vi "Main.vi"() -> ()   [LabVIEW 2017, in "Client.lvlib"]
uses:
  Client.lvlib
  UI_API/UIReferences.ctl
  UI_API/SR Fields.ctl
  ParserSorter/SR Data.ctl
  ParserSorter/AE Group.ctl
  ParserSorter/SR Status.ctl
  ParserSorter/SR Level.ctl
  ParserSorter/SR Type.ctl
  ServerCommunications/TypeDefs/Connection Status.ctl
  CommunicationsFrameWork/TypeDefs/InternalData.ctl
  ServerCommunications/TypeDefs/SR List.ctl
  ServerCommunications/TypeDefs/SR Data.ctl
  ClientErrorHandler/ErrorLoopInitData.ctl
  CommunicationsFrameWork/CommsFrameWork.lvlib
  ServerCommunications/CommsServer.lvlib
  <vilib>/httpClient/LabVIEWHTTPClient.lvlib
  ClientErrorHandler/ClientErrorHandler.lvlib
  ClientLogger/ClientLogger.lvlib
  ParserSorter/ParserSorter.lvlib
  UI_API/UI_API.lvlib
panel:
  in  "Filter Preset":enum16{"All", "Eastern Europe", "DACH"}(ring)
  out "Time to Refresh":dbl(slide) scale=0.0..10.0
  in  "Stop":bool
  out "Connection Quality":dbl(knob) scale=0.0..10.0
  out "Connected?":bool
  out "Last Update":timestamp
  in  "Refresh":bool
  in  "AE Level":enum16{"AE / ELP", "AE Intern"}(ring)
  in  "AE Groups":i32[](listbox)
  in  "SRs Tab":enum32{"Unassigned", "Assigned", "Debug"}(tab)
  out "Unassigned Sorted SRs":string[][](table)
  out "Assigned Sorted SRs":string[][](table)
  out "Last Error":errorcluster
  in  "Text":string="Manual Log Entry"
  in  "Type":string="Event"
  in  "Generate Log Entry":bool
  in  "Injected Error":errorcluster
  in  "Generate Error":bool
  out "Header":string="HTTP/1.1 200 OK\r\nConnection: Keep-Alive\r\nServer: Embedthis-http\r\nContent-Type: text/xml; charset=utf-8\r\nCache-Control: no-cache\r\nDate: Fri, 26 Jan 2018 14:34:54 GMT\r\nContent-Length: 21\r\nKeep-Alive: timeout=60, max=199\r\n\r\n"
  out "Body":string="<Response></Response>"
  in  "DecorationControl":i32(listbox)
  # "Heartbeat Communication"
  # "Manual Loop Control"
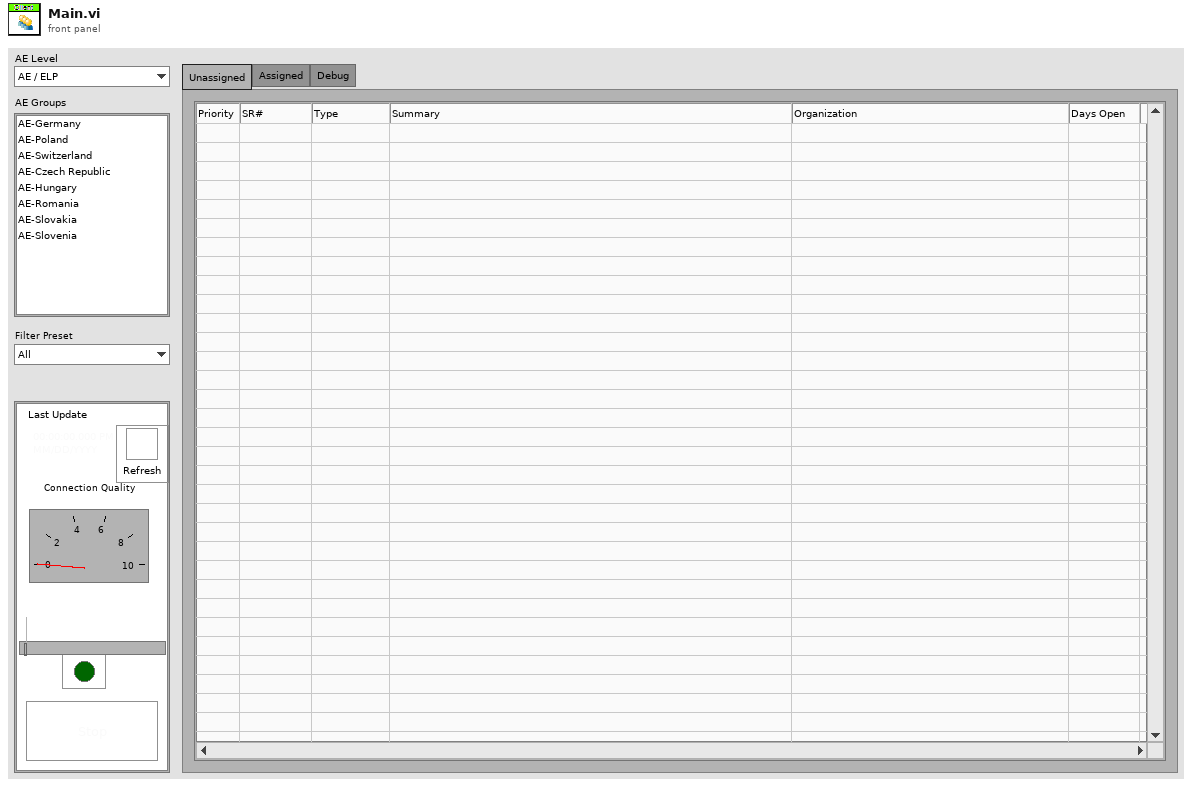
[diagram p1: front panel]
types:
  T1 = typedef "Client.lvlib/CommsFrameWork.lvlib/CommReferences.ctl" = cluster{"ErrorEventReg":refnum<event-registration>, "ErrorEvent":refnum<user-event>, "Queues":cluster{"MHLClient":refnum<queue>, "ErrorHandler":refnum<queue>, "EventHandler":refnum<queue>, "ConnectionHandler":refnum<queue>, "UIHandler":refnum<queue>, "Logger":refnum<queue>}}
  T2 = typedef "LVPoint32TypeDef.ctl" = cluster{"Horizontal":i32, "Vertical":i32}
  T3 = typedef "Client.lvlib/UI_API.lvlib/UIReferences.ctl" = cluster{"Assigned SRs":refnum<vi>, "Unassigned SRs":refnum<vi>, "AE Level":refnum<vi>, "AE Groups":refnum<vi>}
  T4 = typedef "Client.lvlib/ParserSorter.lvlib/SR Data.ctl" = cluster{"SR Number":i64, "AE Group":T5, "SR Owner":string, "Summary":string, "SR Status":T6, "Days Open":dbl, "Prio":T7, "SR Type":T8, "Service Level":string, "Last Updated":timestamp, "First Name":string, "Last Name":string, "Organisation Name":string, "Creation Date":timestamp, "Needs Merging?":bool, "English Flag?":bool}
  T5 = typedef "Client.lvlib/ParserSorter.lvlib/AE Group.ctl" = enum32{"NaN", "AE-Germany", "AE-Poland", "AE-Switzerland", "AE-Czech Republic", "AE-Hungary", "AE-Romania", "AE-Slovakia", "AE-Slovenia"}
  T6 = typedef "Client.lvlib/ParserSorter.lvlib/SR Status.ctl" = enum32{"NaN", "Caller Abandoned", "Created in Error", "Declined to Purchase Support", "Expired", "Forum Resolved AE", "Forum Resolved Customer", "IN WORK", "IN WORK Collab with AES", "IN WORK Collab with PSE", "IN WORK Collab with SE", "IN WORK Escalation", "IN WORK Customer Added Note", "Open", "Potentially Resolved", "POC Resolved", "Resolved", "RMA Waiting on Customer", "RMA Open", "RMA In Progress", "RMA Closed - DOA", "RMA Closed", "RMA Approved for Return", "Project Complete", "Presumed Resolved", "IN WORK Wait on Customer"}
  T7 = typedef "Client.lvlib/ParserSorter.lvlib/SR Level.ctl" = enum16{"Prio 1", "Prio 2", "Prio 3", "Prio 4"}
  T8 = typedef "Client.lvlib/ParserSorter.lvlib/SR Type.ctl" = enum32{"NaN", "ATE Core Configurations (BYOATE)", "Activation", "BioBench", "CAN", "CM C Series", "Calibration", "Consulting Services", "CounterTimer", "DAQExpress", "DASYLab", "DIAdem", "DMM", "DSA HW", "Digital_IO", "FIRST (NIC Only)", "FieldBus", "FieldPoint", "Functional Savety", "GATI", "GPIB", "HMI and Industrial PCs", "HiQ", "HighSpeedDigital_IO", "IMAQ", "IOTech Vibration", "Industrial Communications", "InsightCM", "LV", "LV CD&Sim", "LV Comms", "LV Controls Add-Ons", "LV Embedded", "LV MathScript RT", "LV NXG", "LV NXT", "LVDSC", "LVFPGA", "LVPDA and LV Touch Panel", "LVRT", "LabWindows_CVI", "Lookout", "MATRIXx", "MStudioDotNet", "MStudioVisualBasic", "MStudioVisualC", "Measure (Legacy)", "Motion", "MultifunctionDAQ", "Multimedia Test HW/SW", "Multisim (EWB)", "NI Update Service", "OPC Servers", "Optical (OSI)", "PXI Controllers, Chassis, MXI", "PXI Timing and Sync", "Power Supplies and SMUs", "Powertrain Controls", "RAID", "RF", "RF Software", "RIO", "SC Express", "SCC", "SCXI", "SPEEDY-33 (Hyperception)", "STS", "ScopeDigitizers", "Serial", "Signal Sources", "SignalCondOther", "SignalExpress", "Software Defined Intruments", "Sound and Vibration SW", "Switch Executive", "Switches", "TestStand", "USRP", "Ultiboard (EWB)", "VBench", "VI Logger", "VXI_MXI", "VeriStand", "VisionSW", "VolumeLicenseMgr", "WSN", "Web UI Builder", "myRIO"}
  T9 = typedef "Client.lvlib/CommsServer.lvlib/Connection Status.ctl" = cluster{"Connection Quality":dbl, "Last Update":timestamp}
  T10 = typedef "Client.lvlib/ParserSorter.lvlib/SR Fields.ctl" = enum16{"SR Number", "AE Group", "SR Owner", "Summary", "SR Status", "Days Open", "Prio", "SR Type", "Service Level", "Last Updated", "First Name", "Last Name", "Organisation Name", "Creation Date", "Needs Merging?", "English Flag?"}
  T11 = typedef "Client.lvlib/ClientErrorHandler.lvlib/ErrorLoopInitData.ctl" = cluster{"ErrorsToIgnore":i32[]}
  T12 = typedef "Client.lvlib/CommsFrameWork.lvlib/InternalData.ctl" = cluster{"Connection Data":cluster{"IP":string, "Port":string, "ClientName":string}}
  T13 = typedef "Client.lvlib/CommsServer.lvlib/SR List.ctl" = T14[]
  T14 = typedef "Client.lvlib/CommsServer.lvlib/SR Data.ctl" = cluster{"SR#":dbl, "Group":string, "Owner":string, "Problem Summary":string, "Last Updated":timestamp, "Customer First Name":string, "Customer Last Name":string, "Company":string, "Created On":timestamp, "SR Type":string, "Status":string, "Service Level":string, "Channel":string, "Days Open":dbl}
  T15 = cluster{"IP":string, "Port":string, "ClientName":string}
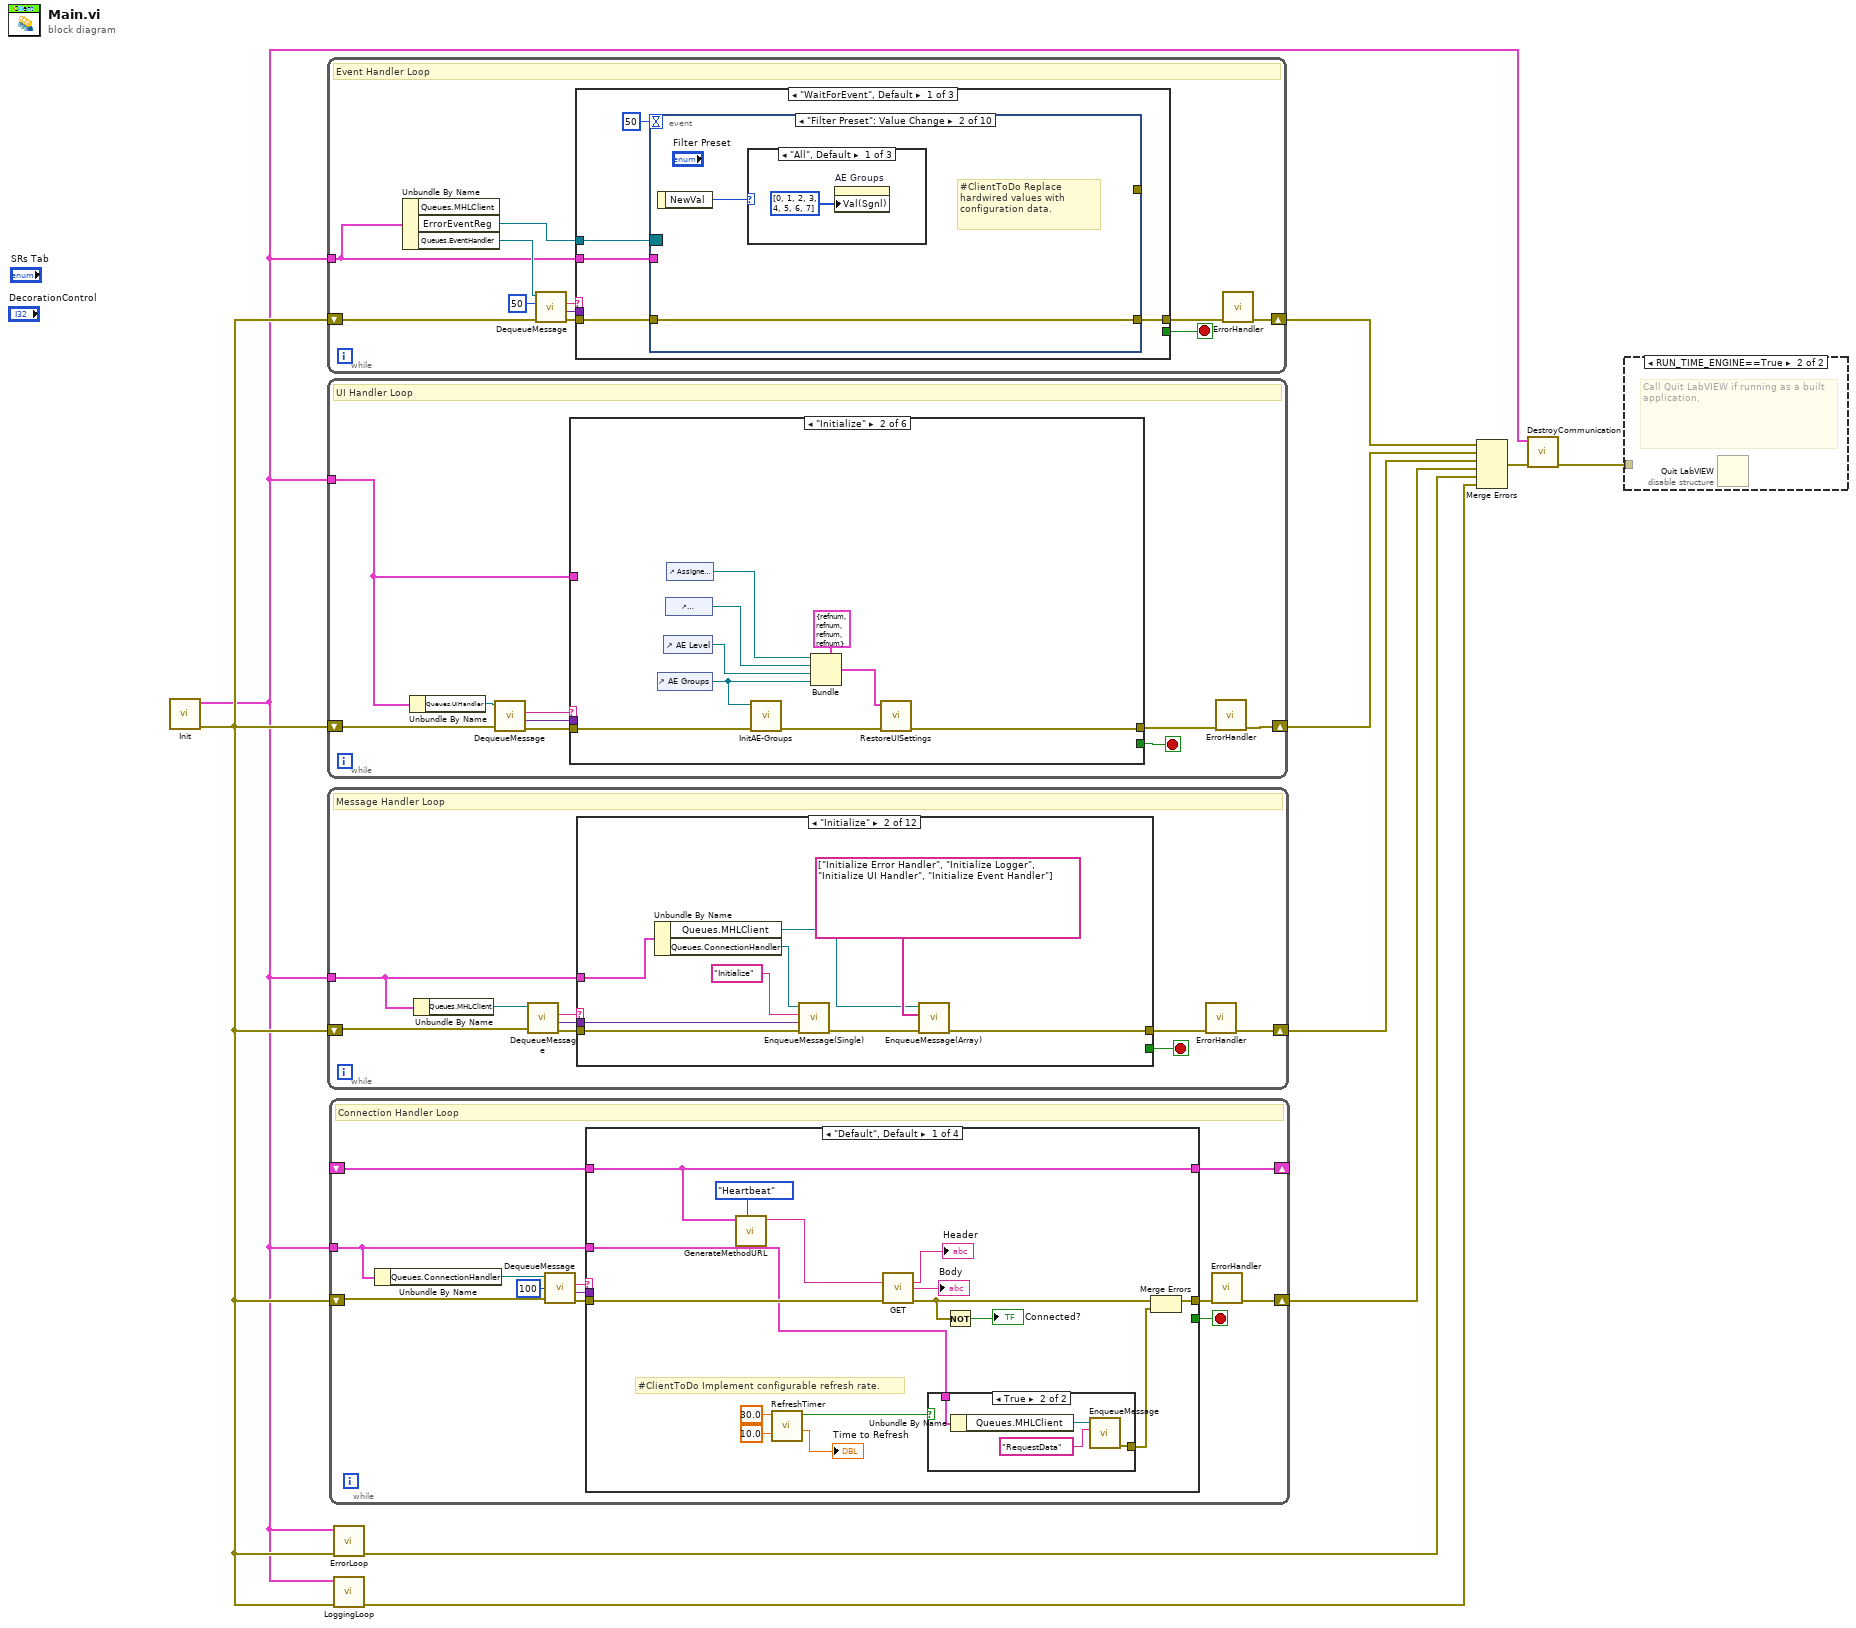
[diagram p0: block diagram]
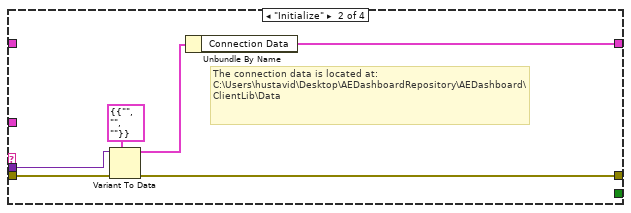
[diagram p4: hidden frame]
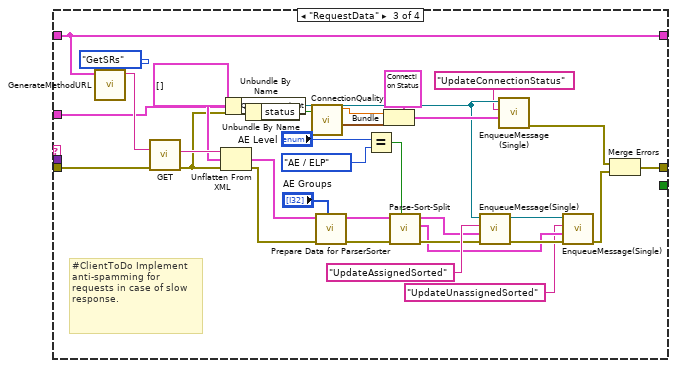
[diagram p5: hidden frame]
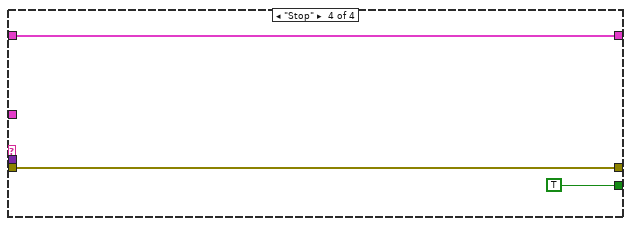
[diagram p6: hidden frame]
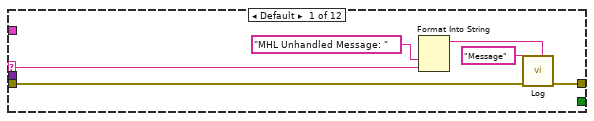
[diagram p7: hidden frame]
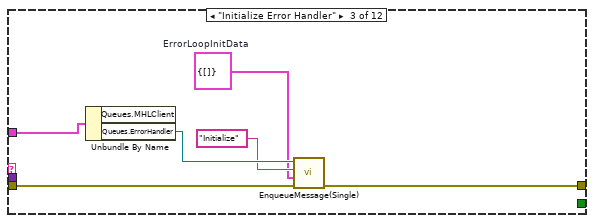
[diagram p8: hidden frame]
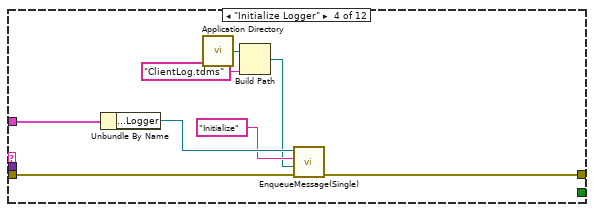
[diagram p9: hidden frame]
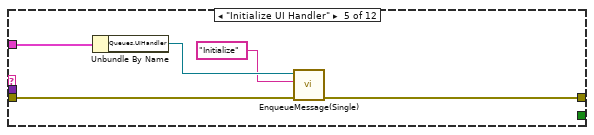
[diagram p10: hidden frame]
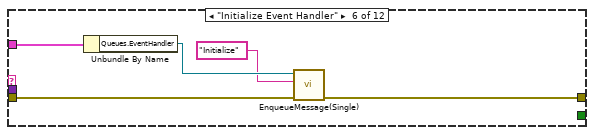
[diagram p11: hidden frame]
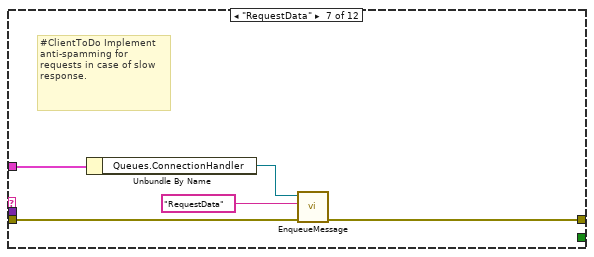
[diagram p12: hidden frame]
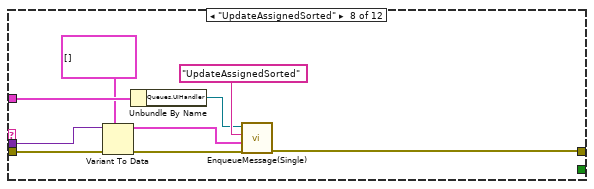
[diagram p13: hidden frame]
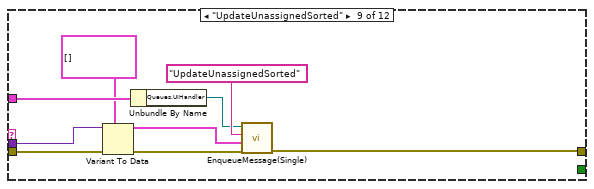
[diagram p14: hidden frame]
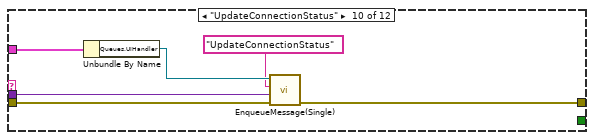
[diagram p15: hidden frame]
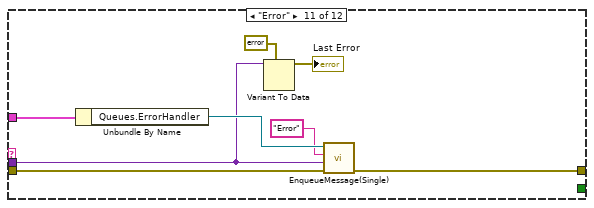
[diagram p16: hidden frame]
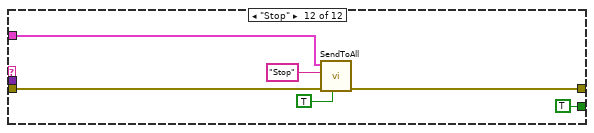
[diagram p17: hidden frame]
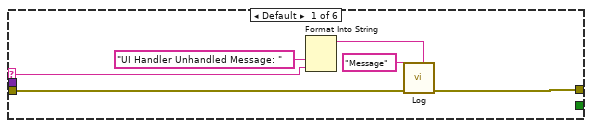
[diagram p18: hidden frame]
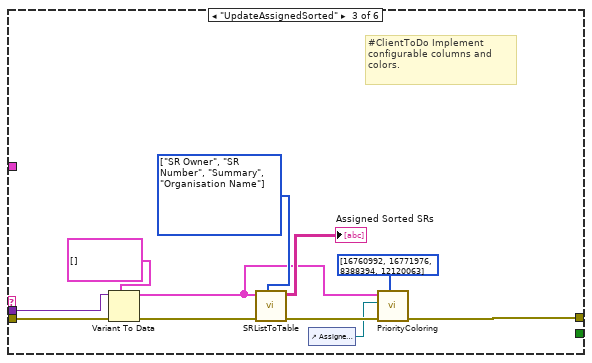
[diagram p19: hidden frame]
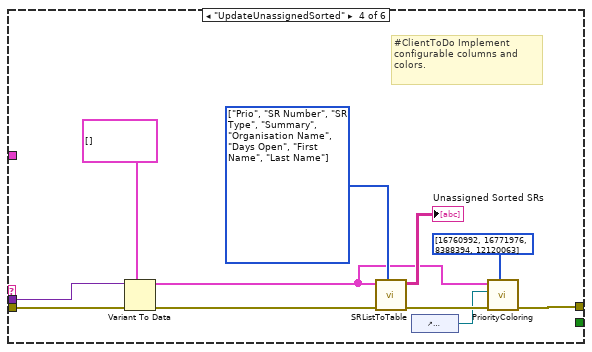
[diagram p20: hidden frame]
diagram:
  n1 = call "Init.vi"() -> ("Error Out"=w4:errorcluster, "Message Queues"=w3:T1)  [unwired: 10 in]
  n2 = while {
    tunnel: w3 -> [w12]
    shift-right: [w13] -> w9
    shift-left: w4 -> [w20]
    stop <- w16 stop-if-true
    # "Event Handler Loop"
    n3 = Unbundle By Name(w12) -> ("ErrorEventReg"=w11:refnum<event-registration>, "Queues.EventHandler"=w21:refnum<queue>)  [unwired: 1 out]
    n4 = call "DequeueMessage.vi"("error in (no error)"=w20, "timeout ms (-1)"=50, "Message Queue"=w21) -> ("error out"=w18:errorcluster, "Message Data"=w17:variant, "Message"=w19:string)  [unwired: 4 in, 2 out]
    n5 = case shown="\"WaitForEvent\", Default" w19 {
      tunnel: w18 -> [w26 w105 w108]
      tunnel: [w23 w104 w108] -> w14
      tunnel: w17 -> [_ _ _]
      tunnel: [_ _ TRUE] -> w16
      tunnel: w12 -> [w25 w103 _]
      tunnel: w11 -> [w22 _ _]
      frame "WaitForEvent", Default {
        n6 = event shown="[1] \"Filter Preset\": Value Change" {
          selector: w22 -> [_ _ _ _ _ _ _ _ _ _]
          dyn-events: _ -> [_ _ _ _ _ _ _ _ _ _]
          timeout: 50 -> [_ _ _ _ _ _ _ _ _ _]
          tunnel: w26 -> [w29 w33 w38 w40 w47 w51 w59 w76 w82 w102]
          tunnel: w25 -> [w31 _ _ _ w46 w53 _ w79 _ w99]
          tunnel: [w30 w33 w38 w39 w43 w50 w58 w77 w81 w101] -> w23
          tunnel: [_ _ _ _ _ w48 _ _ _ _] -> _
          event Timeout {
            n7 = event-data() -> ()  [unwired: 1 in, 3 out]
            n8 = Unbundle By Name(w31) -> ("Queues.EventHandler"=w27:refnum<queue>)
            n9 = call "EnqueueMessage(Single).vi"("error in (no error)"=w29, "Message"="WaitForEvent", "Message Queue"=w27) -> ("error out"=w30:errorcluster)  [unwired: 7 in, 1 out]
          }
          event "Filter Preset": Value Change {
            # "#ClientToDo Replace hardwired values with configuration data."
            n10 = event-data() -> ("NewVal"=w32:enum16{"All", "Eastern Europe", "DACH"})  [unwired: 1 in]
            n11 = case shown="\"All\", Default" w32 {
              frame "All", Default {
                n12 = property on="AE Groups" class="LstBox (strict)"("Val(Sgnl)"=i32[] [0, 1, 2, 3, 4, 5, 6, 7] ("Value (Signaling)")) -> ()  [unwired: 2 in, 2 out]
              }
              frame "Eastern Europe" {
                n13 = property on="AE Groups" class="LstBox (strict)"("Val(Sgnl)"=i32[] [1, 3, 4, 5, 6, 7] ("Value (Signaling)")) -> ()  [unwired: 2 in, 2 out]
              }
              frame "DACH" {
                n14 = property on="AE Groups" class="LstBox (strict)"("Val(Sgnl)"=i32[] [0, 2] ("Value (Signaling)")) -> ()  [unwired: 2 in, 2 out]
              }
            }
          }
          event "Generate Error": Value Change {
            n15 = event-data() -> ()  [unwired: 1 in, 6 out]
            n16 = call "ErrorHandler.vi"("error in (no error)"="Injected Error") -> ()  [unwired: 10 in, 1 out]
          }
          event "Generate Log Entry": Value Change {
            n17 = event-data() -> ()  [unwired: 1 in, 6 out]
            n18 = call "Log.vi"("LogMessage"="Text", "Type"="Type", "Error In"=w40) -> ("Error Out"=w39:errorcluster)  [unwired: 8 in]
          }
          event "Refresh": Value Change {
            n19 = event-data() -> ()  [unwired: 1 in, 1 out]
            n20 = Unbundle By Name(w46) -> ("Queues.MHLClient"=w45:refnum<queue>)
            n21 = call-poly "EnqueueMessage.vi"("error in (no error)"=w47, "Message"="RequestData", "Message Queue"=w45) -> ("error out"=w43:errorcluster)  [unwired: 7 in, 1 out]
          }
          event User Event {
            n22 = event-data() -> ("status"=w56:bool, "code"=w55:i32, "source"=w54:string)  [unwired: 1 in]
            n23 = Unbundle By Name(w53) -> ("Queues.MHLClient"=w52:refnum<queue>)
            n24 = Bundle(cluster=errorcluster {"status"=FALSE, "code"=0, "source"=""} ("error constant"), "status"=w56, "code"=w55, "source"=w54) -> (w48:errorcluster)
            n25 = call "EnqueueMessage(Single).vi"("error in (no error)"=w51, "Message"="Stop", "Message Queue"=w52) -> ("error out"=w50:errorcluster)  [unwired: 7 in, 1 out]
          }
          event "Unassigned Sorted SRs": Shortcut Menu Selection (User) {
            # "#ClientToDo Adapt SR# finding to configurable columns"
            n26 = event-data() -> ("ItemTag"=w60:string, "CtlRef"=w62:refnum<vi>, "Coords"=w61:T2)  [unwired: 1 in]
            n27 = case shown="\"Copy SR#\", Default" w60 {
              tunnel: w62 -> [w68 w73]
              tunnel: w61 -> [w67 w71]
              tunnel: [w63 w70] -> w58
              tunnel: w59 -> [w64 w69]
              frame "Open Screenpop" {
                # "#ClientToDo URL from config data."
                n28 = call "Open Screenpop.vi"("Screenpop URL Prefix"="http://force.natinst.com:8000/pls/ebiz/niae_screenpop.main?p_incident_number=", "SR# Cloumn Header"="SR#" ("SR Cloumn Header"), "Error In"=w64, "Coordinates"=w67, "Table Reference"=w68) -> ("Error Out"=w63:errorcluster)  [unwired: 6 in]
              }
              frame "Copy SR#", Default {
                n29 = call "Copy SR Num to Clipboard.vi"("SR Cloumn Header"="SR#", "Error In"=w69, "Coordinates"=w71, "Table Reference"=w73) -> ("Error Out"=w70:errorcluster)  [unwired: 7 in]
              }
            }
          }
          event Panel Close? {
            n30 = event-data() -> ()  [unwired: 1 in, 1 out]
            n31 = Unbundle By Name(w79) -> ("Queues.MHLClient"=w78:refnum<queue>)
            n32 = call "EnqueueMessage(Single).vi"("Priority Message? (F)"=TRUE, "error in (no error)"=w76, "Message"="Stop", "Message Queue"=w78) -> ("error out"=w77:errorcluster)  [unwired: 6 in, 1 out]
            n33 = event-data("Discard?"=TRUE) -> ()  [unwired: 1 in, 1 out]
          }
          event "Assigned Sorted SRs": Shortcut Menu Selection (User) {
            # "#ClientToDo Adapt SR# finding to configurable columns"
            n34 = event-data() -> ("ItemTag"=w85:string, "CtlRef"=w84:refnum<vi>, "Coords"=w83:T2)  [unwired: 1 in]
            n35 = case shown="\"Open Screenpop\"" w85 {
              tunnel: w84 -> [w91 w96]
              tunnel: w83 -> [w90 w94]
              tunnel: w82 -> [w87 w93]
              tunnel: [w86 w92] -> w81
              frame "Open Screenpop" {
                # "#ClientToDo URL from config data."
                n36 = call "Open Screenpop.vi"("Screenpop URL Prefix"="http://force.natinst.com:8000/pls/ebiz/niae_screenpop.main?p_incident_number=", "SR# Cloumn Header"="SR#" ("SR Cloumn Header"), "Error In"=w87, "Coordinates"=w90, "Table Reference"=w91) -> ("Error Out"=w86:errorcluster)  [unwired: 6 in]
              }
              frame "Copy SR#", Default {
                n37 = call "Copy SR Num to Clipboard.vi"("SR Cloumn Header"="SR#", "Error In"=w93, "Coordinates"=w94, "Table Reference"=w96) -> ("Error Out"=w92:errorcluster)  [unwired: 7 in]
              }
            }
          }
          event "Stop": Value Change {
            n38 = event-data() -> ()  [unwired: 1 in, 1 out]
            n39 = Unbundle By Name(w99) -> ("Queues.MHLClient"=w100:refnum<queue>)
            n40 = call-poly "EnqueueMessage.vi"("Priority Message? (F)"=TRUE, "error in (no error)"=w102, "Message"="Stop", "Message Queue"=w100) -> ("error out"=w101:errorcluster)  [unwired: 6 in, 1 out]
          }
        }
      }
      frame "Initialize" {
        n41 = Unbundle By Name(w103) -> ("Queues.EventHandler"=w107:refnum<queue>)
        n42 = call "EnqueueMessage(Single).vi"("error in (no error)"=w105, "Message"="WaitForEvent", "Message Queue"=w107) -> ("error out"=w104:errorcluster)  [unwired: 7 in, 1 out]
      }
      frame "Stop" {
      }
    }
    n43 = call "ErrorHandler.vi"("error in (no error)"=w14) -> ("error out"=w13:errorcluster)  [unwired: 10 in]
  }
  n44 = while {
    tunnel: w3 -> [w112]
    shift-right: [w110] -> w8
    shift-left: w4 -> [w117]
    stop <- w113 stop-if-true
    # "UI Handler Loop"
    n45 = Unbundle By Name(w112) -> ("Queues.UIHandler"=w118:refnum<queue>)
    n46 = call "DequeueMessage.vi"("error in (no error)"=w117, "Message Queue"=w118) -> ("error out"=w116:errorcluster, "Message Data"=w114:variant, "Message"=w115:string)  [unwired: 5 in, 2 out]
    n47 = case shown="\"Initialize\"" w115 {
      selector: w115 -> [w121 _ _ _ _ _]
      tunnel: w116 -> [w120 w133 w143 w151 w162 w164]
      tunnel: [w119 w126 w137 w148 w161 w163] -> w111
      tunnel: w114 -> [_ _ w144 w152 w160 _]
      tunnel: [_ _ _ _ _ TRUE] -> w113
      tunnel: w112 -> [_ _ _ _ _ _]
      frame Default {
        n48 = Format Into String("UI Handler Unhandled Message: " ("Type"), w121) -> (resulting string=w124:string)  [unwired: 3 in, 1 out]
        n49 = call "Log.vi"("LogMessage"=w124, "Type"="Message", "Error In"=w120) -> ("Error Out"=w119:errorcluster)  [unwired: 8 in]
      }
      frame "Initialize" {
        n50 = control-ref of="AE Groups"() -> (w128:refnum<vi>)
        n51 = control-ref of="AE Level"() -> (w130:refnum<vi>)
        n52 = control-ref of="Unassigned Sorted SRs"() -> (w131:refnum<vi>)
        n53 = control-ref of="Assigned Sorted SRs"() -> (w132:refnum<vi>)
        n54 = call "InitAE-Groups.vi"("Error In"=w133, "LstBox Refnum"=w128) -> ("Error Out"=w127:errorcluster)  [unwired: 9 in]
        n55 = Bundle(cluster=T3 {"Assigned SRs"=refnum, "Unassigned SRs"=refnum, "AE Level"=refnum, "AE Groups"=refnum} ("UI References"), "Assigned SRs"=w132, "Unassigned SRs"=w131, "AE Level"=w130, "AE Groups"=w128) -> (w125:T3)
        n56 = call "RestoreUISettings.vi"("Error In"=w127, "UI References"=w125) -> ("Error Out"=w126:errorcluster)  [unwired: 9 in]
      }
      frame "UpdateAssignedSorted" {
        w140 = T10[] [enum."SR Owner", enum."SR Number", enum."Summary", enum."Organisation Name"] items=["SR Number", "AE Group", "SR Owner", "Summary", "SR Status", "Days Open", "Prio", "SR Type", "Service Level", "Last Updated", "First Name", "Last Name", "Organisation Name", "Creation Date", "Needs Merging?", "English Flag?"] ("Fields to include")
        # "#ClientToDo Implement configurable columns and colors."
        n57 = Variant To Data(error in=w143, type=T4[] [] ("SR List In"), Variant=w144) -> (data=w135:T4[], error out=w142:errorcluster)
        n58 = call "SRListToTable.vi"("Fields to include"=w140, "Error In"=w142, "SR List In"=w135) -> ("Error Out"=w138:errorcluster, "2D String Array for Table"=→"Assigned Sorted SRs":string[][])  [unwired: 7 in]
        n59 = control-ref of="Assigned Sorted SRs"() -> (w134:refnum<vi>)
        n60 = call "PriorityColoring.vi"("Array"=u32[] [16760992, 16771976, 8388394, 12120063], "Error In"=w138, "Tbl Refnum"=w134, "SR List In"=w135) -> ("Error Out"=w137:errorcluster)  [unwired: 7 in]
      }
      frame "UpdateUnassignedSorted" {
        w153 = T10[] [enum."Prio", enum."SR Number", enum."SR Type", enum."Summary", enum."Organisation Name", enum."Days Open", enum."First Name", enum."Last Name"] items=["SR Number", "AE Group", "SR Owner", "Summary", "SR Status", "Days Open", "Prio", "SR Type", "Service Level", "Last Updated", "First Name", "Last Name", "Organisation Name", "Creation Date", "Needs Merging?", "English Flag?"] ("Fields to include")
        # "#ClientToDo Implement configurable columns and colors."
        n61 = Variant To Data(error in=w151, type=T4[] [] ("SR List In"), Variant=w152) -> (data=w147:T4[], error out=w155:errorcluster)
        n62 = call "SRListToTable.vi"("Fields to include"=w153, "Error In"=w155, "SR List In"=w147) -> ("Error Out"=w149:errorcluster, "2D String Array for Table"=→"Unassigned Sorted SRs":string[][])  [unwired: 7 in]
        n63 = control-ref of="Unassigned Sorted SRs"() -> (w146:refnum<vi>)
        n64 = call "PriorityColoring.vi"("Array"=u32[] [16760992, 16771976, 8388394, 12120063], "Error In"=w149, "Tbl Refnum"=w146, "SR List In"=w147) -> ("Error Out"=w148:errorcluster)  [unwired: 7 in]
      }
      frame "UpdateConnectionStatus" {
        n65 = Variant To Data(error in=w162, type=T9 {"Connection Quality"=0.0, "Last Update"=timestamp(0 s since 1904-01-01)} ("Connection Status"), Variant=w160) -> (data=w158:T9, error out=w161:errorcluster)
        n66 = Unbundle(w158) -> ("Connection Quality"=→"Connection Quality":dbl, "Last Update"=→"Last Update":timestamp)
      }
      frame "Stop" {
        n67 = control-ref of="AE Groups"() -> (w167:refnum<vi>)
        n68 = control-ref of="AE Level"() -> (w168:refnum<vi>)
        n69 = control-ref of="Unassigned Sorted SRs"() -> (w169:refnum<vi>)
        n70 = control-ref of="Assigned Sorted SRs"() -> (w170:refnum<vi>)
        n71 = Bundle(cluster=T3 {"Assigned SRs"=refnum, "Unassigned SRs"=refnum, "AE Level"=refnum, "AE Groups"=refnum} ("UI References"), "Assigned SRs"=w170, "Unassigned SRs"=w169, "AE Level"=w168, "AE Groups"=w167) -> (w165:T3)
        n72 = call "SaveUISettings.vi"("Error In"=w164, "UI References"=w165) -> ("Error Out"=w163:errorcluster)  [unwired: 9 in]
      }
    }
    n73 = call "ErrorHandler.vi"("error in (no error)"=w111) -> ("error out"=w110:errorcluster)  [unwired: 10 in]
  }
  n74 = while {
    tunnel: w3 -> [w174]
    shift-right: [w172] -> w7
    shift-left: w4 -> [w180]
    stop <- w175 stop-if-true
    # "Message Handler Loop"
    n75 = Unbundle By Name(w174) -> ("Queues.MHLClient"=w179:refnum<queue>)
    n76 = call "DequeueMessage.vi"("error in (no error)"=w180, "Message Queue"=w179) -> ("error out"=w176:errorcluster, "Message Data"=w177:variant, "Message"=w178:string)  [unwired: 5 in, 2 out]
    n77 = case shown="\"Initialize\"" w178 {
      selector: w178 -> [w185 _ _ _ _ _ _ _ _ _ _ _]
      tunnel: w177 -> [_ w195 _ _ _ _ _ w231 w240 w246 w251 _]
      tunnel: w176 -> [w182 w192 w200 w208 w213 w218 w224 w230 w239 w248 w253 w260]
      tunnel: [w181 w188 w196 w205 w210 w215 w223 w225 w234 w247 w252 w259] -> w173
      tunnel: [_ _ _ _ _ _ _ _ _ _ _ TRUE] -> w175
      tunnel: w174 -> [_ w194 w201 w209 w214 w219 w222 w233 w242 w245 w256 w258]
      frame Default {
        n78 = Format Into String("MHL Unhandled Message: " ("Type"), w185) -> (resulting string=w183:string)  [unwired: 3 in, 1 out]
        n79 = call "Log.vi"("LogMessage"=w183, "Type"="Message", "Error In"=w182) -> ("Error Out"=w181:errorcluster)  [unwired: 8 in]
      }
      frame "Initialize" {
        n80 = Unbundle By Name(w194) -> ("Queues.MHLClient"=w187:refnum<queue>, "Queues.ConnectionHandler"=w193:refnum<queue>)
        n81 = call "EnqueueMessage(Single).vi"("error in (no error)"=w192, "Message Data"=w195, "Message"="Initialize", "Message Queue"=w193) -> ("error out"=w190:errorcluster)  [unwired: 6 in, 1 out]
        n82 = call "EnqueueMessage(Array).vi"("error in (no error)"=w190, "Message Array"=string[] ["Initialize Error Handler", "Initialize Logger", "Initialize UI Handler", "Initialize Event Handler"], "Message Queue"=w187) -> ("error out"=w188:errorcluster)  [unwired: 7 in, 1 out]
      }
      frame "Initialize Error Handler" {
        w197 = T11 {"ErrorsToIgnore"=[]}  # ErrorLoopInitData
        n83 = Unbundle By Name(w201) -> ("Queues.ErrorHandler"=w199:refnum<queue>)  [unwired: 1 out]
        n84 = call "EnqueueMessage(Single).vi"("error in (no error)"=w200, "Message Data"=w197, "Message"="Initialize", "Message Queue"=w199) -> ("error out"=w196:errorcluster)  [unwired: 6 in, 1 out]
      }
      frame "Initialize Logger" {
        n85 = Unbundle By Name(w209) -> ("Queues.Logger"=w207:refnum<queue>)
        n86 = call <vilib>:"Application Directory.vi"() -> ("Application Directory"=w204:path)
        n87 = Build Path(base path=w204, name or relative path="ClientLog.tdms") -> (appended path=w202:path)
        n88 = call "EnqueueMessage(Single).vi"("error in (no error)"=w208, "Message Data"=w202, "Message"="Initialize", "Message Queue"=w207) -> ("error out"=w205:errorcluster)  [unwired: 6 in, 1 out]
      }
      frame "Initialize UI Handler" {
        n89 = Unbundle By Name(w214) -> ("Queues.UIHandler"=w212:refnum<queue>)
        n90 = call "EnqueueMessage(Single).vi"("error in (no error)"=w213, "Message"="Initialize", "Message Queue"=w212) -> ("error out"=w210:errorcluster)  [unwired: 7 in, 1 out]
      }
      frame "Initialize Event Handler" {
        n91 = Unbundle By Name(w219) -> ("Queues.EventHandler"=w217:refnum<queue>)
        n92 = call "EnqueueMessage(Single).vi"("error in (no error)"=w218, "Message"="Initialize", "Message Queue"=w217) -> ("error out"=w215:errorcluster)  [unwired: 7 in, 1 out]
      }
      frame "RequestData" {
        # "#ClientToDo Implement anti-spamming for requests in case of slow response."
        n93 = Unbundle By Name(w222) -> ("Queues.ConnectionHandler"=w221:refnum<queue>)
        n94 = call-poly "EnqueueMessage.vi"("error in (no error)"=w224, "Message"="RequestData", "Message Queue"=w221) -> ("error out"=w223:errorcluster)  [unwired: 7 in, 1 out]
      }
      frame "UpdateAssignedSorted" {
        n95 = Variant To Data(error in=w230, type=T4[] [] ("SR List In"), Variant=w231) -> (data=w227:T4[], error out=w226:errorcluster)
        n96 = Unbundle By Name(w233) -> ("Queues.UIHandler"=w229:refnum<queue>)
        n97 = call "EnqueueMessage(Single).vi"("error in (no error)"=w226, "Message Data"=w227, "Message"="UpdateAssignedSorted", "Message Queue"=w229) -> ("error out"=w225:errorcluster)  [unwired: 6 in, 1 out]
      }
      frame "UpdateUnassignedSorted" {
        n98 = Variant To Data(error in=w239, type=T4[] [] ("SR List In"), Variant=w240) -> (data=w236:T4[], error out=w235:errorcluster)
        n99 = Unbundle By Name(w242) -> ("Queues.UIHandler"=w238:refnum<queue>)
        n100 = call "EnqueueMessage(Single).vi"("error in (no error)"=w235, "Message Data"=w236, "Message"="UpdateUnassignedSorted", "Message Queue"=w238) -> ("error out"=w234:errorcluster)  [unwired: 6 in, 1 out]
      }
      frame "UpdateConnectionStatus" {
        n101 = Unbundle By Name(w245) -> ("Queues.UIHandler"=w244:refnum<queue>)
        n102 = call "EnqueueMessage(Single).vi"("error in (no error)"=w248, "Message Data"=w246, "Message"="UpdateConnectionStatus", "Message Queue"=w244) -> ("error out"=w247:errorcluster)  [unwired: 6 in, 1 out]
      }
      frame "Error" {
        n103 = Unbundle By Name(w256) -> ("Queues.ErrorHandler"=w255:refnum<queue>)
        n104 = Variant To Data(type=errorcluster {"status"=FALSE, "code"=0, "source"=""} ("error constant"), Variant=w251) -> (data=→"Last Error":errorcluster)  [unwired: 1 in, 1 out]
        n105 = call "EnqueueMessage(Single).vi"("error in (no error)"=w253, "Message Data"=w251, "Message"="Error", "Message Queue"=w255) -> ("error out"=w252:errorcluster)  [unwired: 6 in, 1 out]
      }
      frame "Stop" {
        n106 = call "SendToAll.vi"("Priority Message? (F)"=TRUE, "error in (no error)"=w260, "Message"="Stop", "Message Queues"=w258) -> ("error out"=w259:errorcluster)  [unwired: 7 in]
      }
    }
    n107 = call "ErrorHandler.vi"("error in (no error)"=w173) -> ("error out"=w172:errorcluster)  [unwired: 10 in]
  }
  n108 = while {
    tunnel: w3 -> [w268]
    shift-right: [w263] -> w6
    shift-left: w4 -> [w274]
    shift-right: [w266] -> _
    shift-left: _ -> [w265]
    stop <- w269 stop-if-true
    # "Connection Handler Loop"
    n109 = Unbundle By Name(w268) -> ("Queues.ConnectionHandler"=w273:refnum<queue>)
    n110 = call "DequeueMessage.vi"("error in (no error)"=w274, "timeout ms (-1)"=100, "Message Queue"=w273) -> ("error out"=w270:errorcluster, "Message Data"=w271:variant, "Message"=w272:string)  [unwired: 4 in, 2 out]
    n111 = case shown="\"Default\", Default" w272 {
      tunnel: w271 -> [_ w298 _ _]
      tunnel: w270 -> [w287 w299 w330 w334]
      tunnel: [w280 w296 w322 w334] -> w264
      tunnel: [_ _ _ TRUE] -> w269
      tunnel: w268 -> [w282 _ w326 _]
      tunnel: [w289 w294 w332 w333] -> w266
      tunnel: w265 -> [w289 _ w332 w333]
      frame "Default", Default {
        # "#ClientToDo Implement configurable refresh rate."
        n112 = call "GenerateMethodURL.vi"("Method"=enum16{"Heartbeat", "GetSRs"}."Heartbeat", "TestClientData"=w289) -> ("String"=w286:string)  [unwired: 9 in]
        n113 = call "RefreshTimer.vi"("Ticker Multiplier"=10.0, "Refresh Period [s]"=30.0 ("Refresh Period")) -> ("Time to Next Refresh"=→"Time to Refresh":dbl, "Refresh Now?"=w278:bool)  [unwired: 8 in]
        n114 = call <vilib>:"GET.vi"("url"=w286, "error in (no error)"=w287) -> ("headers"=→"Header":string, "body"=→"Body":string, "error out"=w279:errorcluster)  [unwired: 10 in, 1 out]
        n115 = case shown="True" w278 {
          tunnel: w282 -> [_ w293]
          tunnel: [_ w290] -> w281
          frame False {
          }
          frame True {
            n116 = Unbundle By Name(w293) -> ("Queues.MHLClient"=w292:refnum<queue>)
            n117 = call-poly "EnqueueMessage.vi"("Message"="RequestData", "Message Queue"=w292) -> ("error out"=w290:errorcluster)  [unwired: 8 in, 1 out]
          }
        }
        n118 = Not(x=w279) -> (.not. x?=→"Connected?":bool)
        n119 = Merge Errors(w279, w281) -> (w280:errorcluster)
      }
      frame "Initialize" {
        # "The connection data is located at:\nC:\\Users\\hustavid\\Desktop\\AEDashboardRepository\\AEDashboard\\ClientLib\\Data"
        n120 = Variant To Data(error in=w299, type=T12 {"Connection Data"={"IP"="", "Port"="", "ClientName"=""}} ("InternalData"), Variant=w298) -> (data=w295:T12, error out=w296:errorcluster)
        n121 = Unbundle By Name(w295) -> ("Connection Data"=w294:T15)
      }
      frame "RequestData" {
        # "#ClientToDo Implement anti-spamming for requests in case of slow response."
        n122 = call "GenerateMethodURL.vi"("Method"=enum16{"Heartbeat", "GetSRs"}."GetSRs", "TestClientData"=w332) -> ("String"=w329:string)  [unwired: 9 in]
        n123 = call <vilib>:"GET.vi"("url"=w329, "error in (no error)"=w330) -> ("body"=w328:string, "error out"=w308:errorcluster)  [unwired: 10 in, 2 out]
        n124 = Unflatten From XML(xml string=w328, type=T13 [] ("SRList"), error in (no error)=w308) -> (value=w325:T13, error out=w324:errorcluster)
        n125 = Unbundle By Name(w326) -> ("Queues.MHLClient"=w301:refnum<queue>)
        n126 = Unbundle By Name(w308) -> ("status"=w307:bool)
        n127 = call "ConnectionQuality.vi"("Error?"=w307) -> ("Last Update"=w303:timestamp, "Connection Quality"=w304:dbl)  [unwired: 9 in]
        n128 = call "Prepare Data for ParserSorter.vi"("AE Groups to Include"="AE Groups", "Error In"=w324, "SRList"=w325) -> ("Error Out"=w320:errorcluster, "Prepared SR List"=w321:T4[])  [unwired: 7 in]
        n129 = Equal?(x="AE Level", y=enum16{"AE / ELP", "AE Intern"}."AE / ELP") -> (x = y?=w318:bool)
        n130 = Bundle(cluster=T9 {"Connection Quality"=0.0, "Last Update"=timestamp(0 s since 1904-01-01)} ("Connection Status"), "Connection Quality"=w304, "Last Update"=w303) -> (w302:T9)
        n131 = call "Parse-Sort-Split.vi"("Include High Priority?"=w318, "Error In"=w320, "SR List In"=w321) -> ("Error Out"=w315:errorcluster, "Unassigned SR List"=w312:T4[], "Assigned SR List"=w316:T4[])  [unwired: 6 in]
        n132 = call "EnqueueMessage(Single).vi"("error in (no error)"=w315, "Message Data"=w316, "Message"="UpdateAssignedSorted", "Message Queue"=w301) -> ("error out"=w314:errorcluster, "dup Message Queue"=w310:refnum<queue>)  [unwired: 6 in]
        n133 = call "EnqueueMessage(Single).vi"("Message Data"=w302, "Message"="UpdateConnectionStatus", "Message Queue"=w301) -> ("error out"=w306:errorcluster)  [unwired: 7 in, 1 out]
        n134 = call "EnqueueMessage(Single).vi"("error in (no error)"=w314, "Message Data"=w312, "Message"="UpdateUnassignedSorted", "Message Queue"=w310) -> ("error out"=w313:errorcluster)  [unwired: 6 in, 1 out]
        n135 = Merge Errors(w306, w313) -> (w322:errorcluster)
      }
      frame "Stop" {
      }
    }
    n136 = call "ErrorHandler.vi"("error in (no error)"=w264) -> ("error out"=w263:errorcluster)  [unwired: 10 in]
  }
  n137 = call "ErrorLoop.vi"("Error In"=w4, "Message Queues"=w3) -> ("Error Out"=w5:errorcluster)  [unwired: 9 in]
  n138 = call "LoggingLoop.vi"("Error In"=w4, "Communication References"=w3) -> ("Error Out"=w2:errorcluster)  [unwired: 9 in]
  n139 = Merge Errors(w9, w8, w7, w6, w5, w2) -> (w10:errorcluster)
  n140 = call "DestroyCommunication.vi"("error in (no error)"=w10, "Message Queues"=w3) -> ("error out"=w1:errorcluster)  [unwired: 9 in]
  n141 = disable-structure shown="RUN_TIME_ENGINE==True" {
    disable-tunnel: w1 -> [_ _]
    frame condition #0 (active) {
    }
    frame condition #1 {
      # "Call Quit LabVIEW if running as a built application."
      n142 = Quit LabVIEW() -> ()  [unwired: 1 in]
    }
  }
